vi "Core_Disconnect.vi"(8 "error in (no error)":errorcluster, 11 "HSMS Class in":refnum<class "HSMS Class.lvclass">) -> (0 "error out":errorcluster, 3 "HSMS Class out":refnum<class "HSMS Class.lvclass">)   [LabVIEW 2020, in "SECS Communication.lvlib" / "HSMS Class.lvclass"]
uses:
  HSMS Class.lvclass
  HSMS Class.lvclass/HSMS Class.ctl
  Notifier Type.ctl
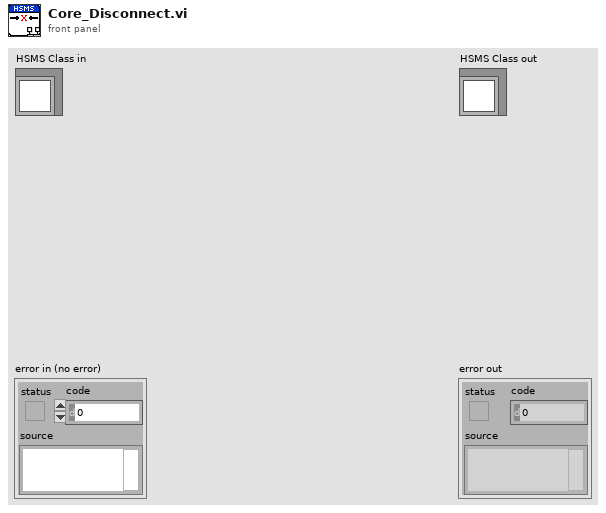
[diagram p1: front panel]
types:
  T1 = typedef "SECS Communication.lvlib/HSMS Class.lvclass/Notifier Type.ctl" = enum16{"TCPIP Connect", "TCPIP Disconnect", "Receive Message", "Send Message", "T3 Timeout", "T6 Timeout", "T7 Timeout", "Error", "Stop"}
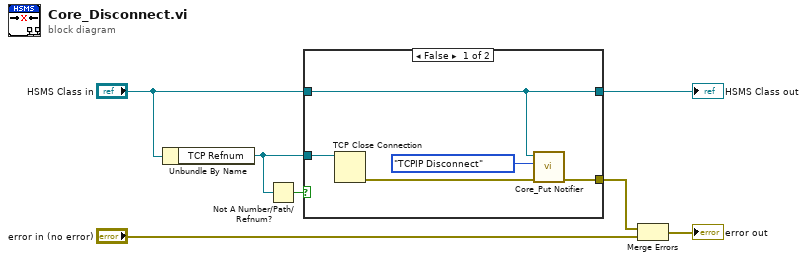
[diagram p0: block diagram]
diagram:
  n1 = Unbundle By Name("HSMS Class in") -> ("TCP Refnum"=w6:refnum<k5>)
  n2 = Not A Number/Path/Refnum?(number/path/refnum=w6) -> (NaN/Path/Refnum?=w7:bool)
  n3 = case shown="False" w7 {
    tunnel: w6 -> [w12 _]
    tunnel: "HSMS Class in" -> [w8 w13]
    tunnel: [w9 _] -> w4
    tunnel: [w8 w13] -> w3
    frame False {
      n4 = TCP Close Connection(connection ID=w12) -> (error out=w10:errorcluster)  [unwired: 2 in, 1 out]
      n5 = call "Core_Put Notifier.vi"("error in (no error)"=w10, "Notifier Type"=Notifier_Type."TCPIP Disconnect", "HSMS Class in"=w8) -> ("error out"=w9:errorcluster)  [unwired: 7 in, 1 out]
    }
    frame True {
    }
  }
  "HSMS Class out" <- w3
  n6 = Merge Errors(w4, "error in (no error)") -> (→"error out":errorcluster)
